vi "Error Test.vi"   [LabVIEW 2012]
uses:
  Non-User VIs/Controls/Device ID.ctl
  User Controls/Array Dimensions.ctl
  Non-User VIs/Error Checking/Set Quiet Mode Functional Global.vi
  Non-User VIs/Error Checking/View Error Log Mode Functional Global.vi
  Non-User VIs/Allocate Memory/AllocateMemory_32f.vi
  Non-User VIs/Error Checking/Add Error Functional Global.vi
  OpenCLV x64.lvlib
types:
  T1 = typedef "Array Dimensions.ctl" = cluster{"Depth":u64, "Height":u64, "Width":u64}
  T2 = typedef "OpenCLV x64.lvlib/Device ID.ctl" = u64
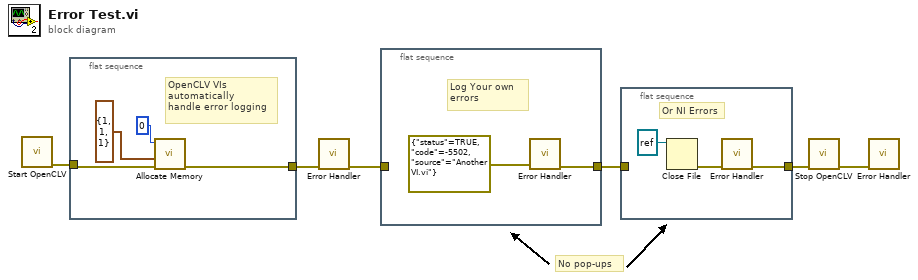
[diagram p0: block diagram]
diagram:
  # "No pop-ups"
  n1 = call "Start OpenCLV.vi"() -> ("Error Out"=w5:errorcluster)  [unwired: 11 in]
  n2 = flat-sequence {
    tunnel: [w10] -> w6
    tunnel: w5 -> [w9]
    frame #0 {
      # "OpenCLV VIs\nautomatically\nhandle error logging"
      n3 = call-poly "Allocate Memory.vi"("Error In"=w9, "Dimension"=T1 {"Depth"=1, "Height"=1, "Width"=1}, "Device In"=T2 0) -> ("Error Out"=w10:errorcluster)  [unwired: 6 in, 2 out]
    }
  }
  n4 = call-poly "Error Handler.vi"("Error In"=w6) -> ("Error Out"=w4:errorcluster)  [unwired: 10 in]
  n5 = flat-sequence {
    tunnel: [w11] -> w3
    tunnel: w4 -> [_]
    frame #0 {
      # "Log Your own \nerrors"
      n6 = call-poly "Error Handler.vi"("Error In"=errorcluster {"status"=TRUE, "code"=-5502, "source"="Another VI.vi"}) -> ("Error Out"=w11:errorcluster)  [unwired: 10 in]
    }
  }
  n7 = flat-sequence {
    tunnel: [w15] -> w2
    tunnel: w3 -> [_]
    frame #0 {
      # "Or NI Errors"
      n8 = Close File(refnum=refnum<file> refnum) -> (error out=w14:errorcluster)  [unwired: 1 in, 1 out]
      n9 = call-poly "Error Handler.vi"("Error In"=w14) -> ("Error Out"=w15:errorcluster)  [unwired: 10 in]
    }
  }
  n10 = call "Stop OpenCLV.vi"("Error In"=w2) -> ("Error Out"=w1:errorcluster)  [unwired: 10 in]
  n11 = call-poly "Error Handler.vi"("Error In"=w1) -> ()  [unwired: 10 in, 1 out]
